vi "Sensor Data Collection.vi"() -> ()   [LabVIEW 2015]
uses:
  Global Variables/refnum names.vi
  Global Variables/Sensor Data.vi
panel:
  in  "Read Enable":T1={"Cal Status"=TRUE, "Orientation"=TRUE, "Gyro"=TRUE, "Accelerometer"=TRUE, "Quaternion"=TRUE, "Accel Mode"=enum."Linear", "Magnetometer"=TRUE}
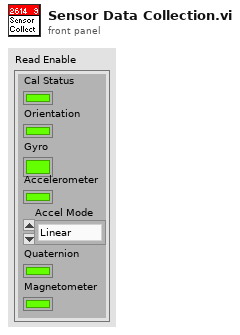
[diagram p1: front panel]
types:
  T1 = cluster{"Cal Status":bool, "Orientation":bool, "Gyro":bool, "Accelerometer":bool, "Quaternion":bool, "Accel Mode":enum8{"Raw Data", "Linear", "Gravity"}, "Magnetometer":bool}
  T2 = typedef "WPI_I2CDevRef.ctl" = cluster{"DevStatus":errorcluster, "Device Address":u8, "Handle":i32, "I2C Bus":T3}
  T3 = typedef "i2c_bus.ctl" = enum16{"I2C On-Board", "I2C MXP", "Invalid"}
  T4 = typedef "WPI_PotentiometerDevRef.ctl" = cluster{"DevStatus":errorcluster, "Analog Channel":T5, "Invert Output":bool}
  T5 = typedef "FPGA_AIChannel.ctl" = enum8{"AI 0", "AI 1", "AI 2", "AI 3", "AI MXP 0", "AI MXP 1", "AI MXP 2", "AI MXP 3", "Invalid"}
  T6 = cluster{"Yaw":dbl, "Roll":dbl, "Pitch":dbl, "Yaw Wind":dbl}
  T7 = typedef "WPI_SwitchDevRef.ctl" = cluster{"DevStatus":errorcluster, "DIO Channel":T8, "CntIndex":T9, "Normally Closed":bool}
  T8 = typedef "FPGA_DIOChannel.ctl" = enum8{"DIO 0", "DIO 1", "DIO 2", "DIO 3", "DIO 4", "DIO 5", "DIO 6", "DIO 7", "DIO 8", "DIO 9", "DIO MXP 0", "DIO MXP 1", "DIO MXP 2", "DIO MXP 3", "DIO MXP 4", "DIO MXP 5", "DIO MXP 6", "DIO MXP 7", "DIO MXP 8", "DIO MXP 9", "DIO MXP 10", "DIO MXP 11", "DIO MXP 12", "DIO MXP 13", "DIO MXP 14", "DIO MXP 15", "Invalid"}
  T9 = typedef "FPGA_CounterCtrSystemIndex.ctl" = enum8{"Ctr 0", "Ctr 1", "Ctr 2", "Ctr 3", "Ctr 4", "Ctr 5", "Ctr 6", "Ctr 7", "Invalid"}
  T10 = typedef "WPI_GyroDevRef.ctl" = cluster{"DevStatus":errorcluster, "Analog Channel":T5, "Offset":dbl, "Gain (VoltsPerDegree/Second)":dbl, "Gyro Type":enum16{"Analog", "XRS450"}, "Handle":i32, "SPI Bus":T11, "Device Found":bool, "Sample Rate":dbl, "Calibrate On Open":bool}
  T11 = typedef "spi_bus.ctl" = enum16{"SPI On-Board, CS0", "SPI On-Board, CS1", "SPI On-Board, CS2", "SPI On-Board, CS3", "SPI MXP", "Invalid"}
  T12 = typedef "WPI_DigitalInputDevRef.ctl" = cluster{"DevStatus":errorcluster, "DIO Channel":T8}
  T13 = typedef "WPI_MotorControlDeviceRef.ctl" = cluster{"DeviceStatus":errorcluster, "Type":T14, "PWM":cluster{"PWM Channel":T15, "DeadBand":T16}, "CAN":cluster{"Device Number":u8, "Control Mode":T17, "Semaphore":T18, "Max Vout":dbl, "TalonSRX Control Mode":T19}, "Invert":bool}
  T14 = typedef "WPI_MotorControlType.ctl" = enum16{"PWM", "CAN", "CANTalonSRX"}
  T15 = typedef "FPGA_DIOPWMChannel.ctl" = enum8{"PWM 0", "PWM 1", "PWM 2", "PWM 3", "PWM 4", "PWM 5", "PWM 6", "PWM 7", "PWM 8", "PWM 9", "PWM MXP 0", "PWM MXP 1", "PWM MXP 2", "PWM MXP 3", "PWM MXP 4", "PWM MXP 5", "PWM MXP 6", "PWM MXP 7", "PWM MXP 8", "PWM MXP 9", "Invalid"}
  T16 = typedef "WPI_PWMDeadband.ctl" = cluster{"Name":string, "maxPositivePwm":i32, "minPositivePwm":i32, "centerPwm":i32, "maxNegativePwm":i32, "minNegativePwm":i32, "angularRange":u16}
  T17 = typedef "WPI_CANJaguar_ControlMode.ctl" = enum8{"Percent VBus", "Current", "Speed", "Position", "Voltage"}
  T18 = typedef "Semaphore RefNum" = refnum<k1>
  T19 = typedef "WPI_CANTalonSRX_APIControlMode.ctl" = enum8{"Percent VBus", "Speed", "Position", "Slave", "Unchanged / Invalid", "Voltage Compensation", "Current", "Motion Profile"}
  T20 = typedef "WPI_CANTalonSRX_GlobalStatus.ctl" = cluster{"Applied Throttle":dbl, "Module Enabled":bool, "CAN Error":errorcluster, "Closed Loop Error":dbl, "Forward Limit Switch Closed":bool, "Reverse Limit Switch Closed":bool, "Sensor Position":dbl, "Sensor Velocity":dbl, "Current":dbl, "Sticky Fault - Over Temp":bool, "Sticky Fault - Under Voltage":bool, "Sticky Fault - Forward Limit":bool, "Sticky Fault - Reverse Limit":bool, "Sticky Fault - Forward Soft Limit":bool, "Sticky Fault - Reverse Soft Limit":bool, "Brake is Enabled":bool, "Encoder Position":dbl, "Encoder Velocity":dbl, "Encoder Index Count":dbl, "Encoder A Pin State":bool, "Encoder B Pin State":bool, "Encoder Index Pin State":bool, "Analog In":dbl, "Analog In Velocity":dbl, "Temperature (C)":dbl, "Battery Voltage":dbl, "Control 5 Is Supported":bool, "Current Profile Slot Select":dbl, "Pos Div 8":bool, "Vel Div 4":bool, "Pulse Width Position":i32, "Pulse Width Velocity":i32, "Pulse Width Rise To Rise (us)":i32, "Pulse Width Rise To Fall (us)":i32, "Mot Prof Active Is Under Run":bool, "Mot Prof Active Has Under Run":bool, "Mot Prof Active Is Last":bool, "Mot Prof Active Velocity Only":bool, "Mot Prof Active Is Valid":bool, "Mot Prof Buffer Is Full":bool, "Mot Prof Active Profile Slot Select":i32, "Mot Prof NextID":i32, "Mot Prof Count":i32, "Mot Prof Active Velocity":dbl, "Mot Prof Active Position":dbl, "Mot Prof Output Enable":i32}
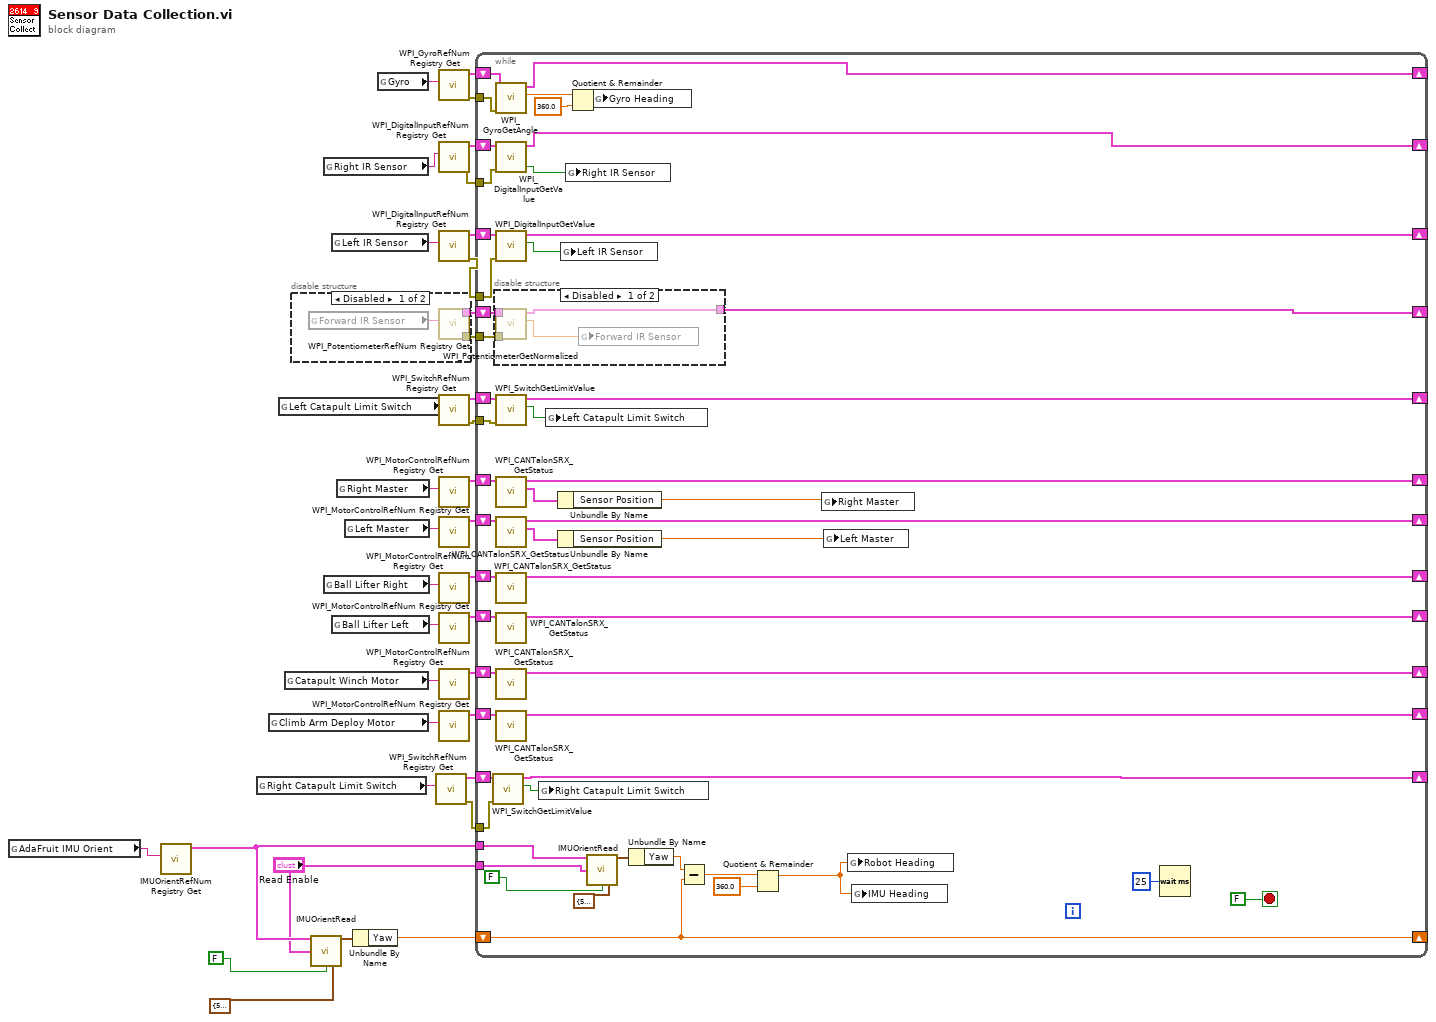
[diagram p0: block diagram]
diagram:
  n1 = global read "refnum names.vi" "AdaFruit IMU Orient"() -> (w7:string)
  n2 = call "IMUOrientRefNum Registry Get.vi"("refnum name"=w7) -> ("I2CDevRef out"=w3:T2)  [unwired: 9 in, 1 out]
  n3 = global read "refnum names.vi" "Right Catapult Limit Switch"() -> (w8:string)
  n4 = global read "refnum names.vi" "Climb Arm Deploy Motor"() -> (w14:string)
  n5 = global read "refnum names.vi" "Left Catapult Limit Switch"() -> (w29:string)
  n6 = global read "refnum names.vi" "Catapult Winch Motor"() -> (w13:string)
  n7 = disable-structure shown="Disabled" {
    disable-tunnel: [w38 _] -> w28
    disable-tunnel: [w37 _] -> w27
    frame Disabled {
      n8 = global read "refnum names.vi" "Forward IR Sensor"() -> (w39:string)
      n9 = call <vilib>:"WPI_PotentiometerRefNum Registry Get.vi"("refnum name"=w39) -> ("error out"=w37:errorcluster, "PotDevRef"=w38:T4)  [unwired: 9 in]
    }
    frame Enabled {
    }
  }
  n10 = call "IMUOrientRead.vi"("I2CDevRef"=w3, "Read Enable"="Read Enable", "Gyro Reset"=FALSE, "Earth Field (uT)"=cluster{"Earth":dbl, "Tolerance":dbl} {"Earth"=51.0, "Tolerance"=5.0}) -> ("Orient Y/R/P"=w4:T6)  [unwired: 5 in, 6 out]
  n11 = global read "refnum names.vi" "Right IR Sensor"() -> (w33:string)
  n12 = global read "refnum names.vi" "Ball Lifter Right"() -> (w18:string)
  n13 = global read "refnum names.vi" "Left IR Sensor"() -> (w32:string)
  n14 = global read "refnum names.vi" "Ball Lifter Left"() -> (w17:string)
  n15 = global read "refnum names.vi" "Right Master"() -> (w20:string)
  n16 = global read "refnum names.vi" "Left Master"() -> (w19:string)
  n17 = Unbundle By Name(w4) -> ("Yaw"=w1:dbl)
  n18 = global read "refnum names.vi" "Gyro"() -> (w36:string)
  n19 = call <vilib>:"WPI_SwitchRefNum Registry Get.vi"("refnum name"=w8) -> ("error out"=w9:errorcluster, "SwitchDevRef"=w10:T7)  [unwired: 9 in]
  n20 = call <vilib>:"WPI_GyroRefNum Registry Get.vi"("refnum name"=w36) -> ("error out"=w35:errorcluster, "GyroDevRef"=w34:T10)  [unwired: 9 in]
  n21 = call <vilib>:"WPI_DigitalInputRefNum Registry Get.vi"("refnum name"=w33) -> ("error out"=w25:errorcluster, "DigitalInputDevRef"=w31:T12)  [unwired: 9 in]
  n22 = call <vilib>:"WPI_DigitalInputRefNum Registry Get.vi"("refnum name"=w32) -> ("error out"=w26:errorcluster, "DigitalInputDevRef"=w30:T12)  [unwired: 9 in]
  n23 = call <vilib>:"WPI_SwitchRefNum Registry Get.vi"("refnum name"=w29) -> ("error out"=w24:errorcluster, "SwitchDevRef"=w23:T7)  [unwired: 9 in]
  n24 = call <vilib>:"WPI_MotorControlRefNum Registry Get.vi"("refnum name"=w20) -> ("MotorControlDevRef"=w22:T13)  [unwired: 9 in, 1 out]
  n25 = call <vilib>:"WPI_MotorControlRefNum Registry Get.vi"("refnum name"=w19) -> ("MotorControlDevRef"=w21:T13)  [unwired: 9 in, 1 out]
  n26 = call <vilib>:"WPI_MotorControlRefNum Registry Get.vi"("refnum name"=w18) -> ("MotorControlDevRef"=w16:T13)  [unwired: 9 in, 1 out]
  n27 = call <vilib>:"WPI_MotorControlRefNum Registry Get.vi"("refnum name"=w17) -> ("MotorControlDevRef"=w15:T13)  [unwired: 9 in, 1 out]
  n28 = call <vilib>:"WPI_MotorControlRefNum Registry Get.vi"("refnum name"=w13) -> ("MotorControlDevRef"=w12:T13)  [unwired: 9 in, 1 out]
  n29 = call <vilib>:"WPI_MotorControlRefNum Registry Get.vi"("refnum name"=w14) -> ("MotorControlDevRef"=w11:T13)  [unwired: 9 in, 1 out]
  n30 = while {
    tunnel: w35 -> [w92]
    shift-right: [w52] -> _
    shift-left: w34 -> [w91]
    shift-right: [w87] -> _
    shift-left: w31 -> [w90]
    shift-right: [w88] -> _
    shift-left: w30 -> [w89]
    shift-right: [w85] -> _
    shift-left: w28 -> [w86]
    tunnel: w27 -> [w84]
    tunnel: w26 -> [w83]
    tunnel: w25 -> [w82]
    tunnel: w24 -> [w81]
    shift-right: [w51] -> _
    shift-left: w23 -> [w80]
    shift-right: [w77] -> _
    shift-left: w22 -> [w79]
    shift-right: [w78] -> _
    shift-left: w21 -> [w76]
    shift-right: [w71] -> _
    shift-left: w16 -> [w75]
    shift-right: [w50] -> _
    shift-left: w15 -> [w74]
    shift-right: [w70] -> _
    shift-left: w12 -> [w73]
    shift-right: [w69] -> _
    shift-left: w11 -> [w72]
    tunnel: w9 -> [w63]
    shift-right: [w65] -> _
    shift-left: w10 -> [w64]
    tunnel: w3 -> [w46]
    tunnel: "Read Enable" -> [w45]
    shift-right: [w43] -> _
    shift-left: w1 -> [w43]
    stop <- FALSE stop-if-true
    n31 = call <vilib>:"WPI_SwitchGetLimitValue.vi"("error in (no error)"=w63, "SwitchDevRef"=w64) -> ("Switch Pressed"=w61:bool, "SwitchDevRef"=w65:T7)  [unwired: 7 in, 1 out]
    n32 = disable-structure shown="Disabled" {
      disable-tunnel: w86 -> [w96 _]
      disable-tunnel: [w95 _] -> w85
      disable-tunnel: w84 -> [w94 _]
      frame Disabled {
        n33 = call <vilib>:"WPI_PotentiometerGetNormalized.vi"("error in"=w94, "PotDevRef"=w96) -> ("Normalized Value"=w93:dbl, "PotDevRef"=w95:T4)  [unwired: 7 in, 1 out]
        n34 = global write "Sensor Data.vi" "Forward IR Sensor"(w93) -> ()
      }
      frame Enabled {
      }
    }
    n35 = call <vilib>:"WPI_GyroGetAngle.vi"("error in"=w92, "GyroDevRef"=w91) -> ("Angle"=w59:dbl, "GyroDevRef"=w52:T10)  [unwired: 5 in, 3 out]
    n36 = call <vilib>:"WPI_DigitalInputGetValue.vi"("error in (no error)"=w82, "DigitalInputDevRef"=w90) -> ("Value"=w67:bool, "DigitalInputDevRef"=w87:T12)  [unwired: 7 in, 1 out]
    n37 = call <vilib>:"WPI_DigitalInputGetValue.vi"("error in (no error)"=w83, "DigitalInputDevRef"=w89) -> ("Value"=w66:bool, "DigitalInputDevRef"=w88:T12)  [unwired: 7 in, 1 out]
    n38 = call <vilib>:"WPI_SwitchGetLimitValue.vi"("error in (no error)"=w81, "SwitchDevRef"=w80) -> ("Switch Pressed"=w60:bool, "SwitchDevRef"=w51:T7)  [unwired: 7 in, 1 out]
    n39 = call <vilib>:"WPI_CANTalonSRX_GetStatus.vi"("CAN Talon SRX Ref"=w79) -> ("Talon SRX Status"=w56:T20, "CAN Talon SRX Ref"=w77:T13)  [unwired: 8 in, 1 out]
    n40 = call <vilib>:"WPI_CANTalonSRX_GetStatus.vi"("CAN Talon SRX Ref"=w76) -> ("Talon SRX Status"=w54:T20, "CAN Talon SRX Ref"=w78:T13)  [unwired: 8 in, 1 out]
    n41 = call <vilib>:"WPI_CANTalonSRX_GetStatus.vi"("CAN Talon SRX Ref"=w75) -> ("CAN Talon SRX Ref"=w71:T13)  [unwired: 8 in, 2 out]
    n42 = call <vilib>:"WPI_CANTalonSRX_GetStatus.vi"("CAN Talon SRX Ref"=w74) -> ("CAN Talon SRX Ref"=w50:T13)  [unwired: 8 in, 2 out]
    n43 = call <vilib>:"WPI_CANTalonSRX_GetStatus.vi"("CAN Talon SRX Ref"=w73) -> ("CAN Talon SRX Ref"=w70:T13)  [unwired: 8 in, 2 out]
    n44 = call <vilib>:"WPI_CANTalonSRX_GetStatus.vi"("CAN Talon SRX Ref"=w72) -> ("CAN Talon SRX Ref"=w69:T13)  [unwired: 8 in, 2 out]
    n45 = global write "Sensor Data.vi" "Right Catapult Limit Switch"(w61) -> ()
    n46 = global write "Sensor Data.vi" "Left Catapult Limit Switch"(w60) -> ()
    n47 = Unbundle By Name(w56) -> ("Sensor Position"=w55:dbl)
    n48 = Unbundle By Name(w54) -> ("Sensor Position"=w53:dbl)
    n49 = global write "Sensor Data.vi" "Left IR Sensor"(w66) -> ()
    n50 = global write "Sensor Data.vi" "Right IR Sensor"(w67) -> ()
    n51 = Quotient & Remainder(x=w59, y=360.0) -> (x-y*floor(x/y)=w57:dbl)  [unwired: 1 out]
    n52 = call "IMUOrientRead.vi"("I2CDevRef"=w46, "Read Enable"=w45, "Gyro Reset"=FALSE, "Earth Field (uT)"=cluster{"Earth":dbl, "Tolerance":dbl} {"Earth"=51.0, "Tolerance"=5.0}) -> ("Orient Y/R/P"=w47:T6)  [unwired: 5 in, 6 out]
    n53 = global write "Sensor Data.vi" "Gyro Heading"(w57) -> ()
    n54 = Unbundle By Name(w47) -> ("Yaw"=w44:dbl)
    n55 = Subtract(x=w44, y=w43) -> (x-y=w42:dbl)
    n56 = Quotient & Remainder(x=w42, y=360.0) -> (x-y*floor(x/y)=w41:dbl)  [unwired: 1 out]
    n57 = global write "Sensor Data.vi" "Right Master"(w55) -> ()
    n58 = global write "Sensor Data.vi" "Left Master"(w53) -> ()
    n59 = global write "Sensor Data.vi" "Robot Heading"(w41) -> ()
    n60 = global write "Sensor Data.vi" "IMU Heading"(w41) -> ()
    n61 = Wait (ms)(milliseconds to wait=u32 25) -> ()  [unwired: 1 out]
  }
